vi "Variant to Reply String.vi"(8 "error in (no error)":errorcluster, 9 "Data":variant, 11 "Instrument.VRM in":refnum<class "Instrument.OxfordVRM.lvclass">) -> (0 "error out":errorcluster, 1 "Reply":string, 3 "Instrument.VRM out":refnum<class "Instrument.OxfordVRM.lvclass">)   [LabVIEW 2019, in "Instrument.OxfordVRM.lvclass"]
uses:
  Instrument.OxfordVRM.lvclass
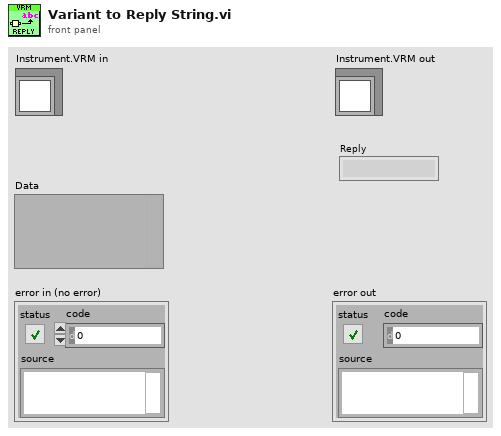
[diagram p1: front panel]
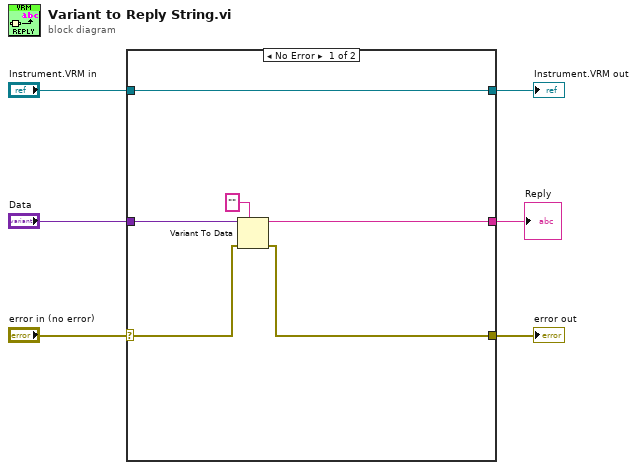
[diagram p0: block diagram]
diagram:
  n1 = case shown="No Error" "error in (no error)" {
    selector: "error in (no error)" -> [w10 w14]
    tunnel: "Data" -> [w9 _]
    tunnel: [w8 w14] -> w5
    tunnel: "Instrument.VRM in" -> [w12 w13]
    tunnel: [w12 w13] -> w2
    tunnel: [w7 _] -> w1
    frame No Error {
      n2 = Variant To Data(error in=w10, type="", Variant=w9) -> (data=w7:string, error out=w8:errorcluster)
    }
    frame Error {
    }
  }
  "Instrument.VRM out" <- w2
  "error out" <- w5
  "Reply" <- w1
